vi "Is_it_a_Results_File.vi"(0 "character string":string) -> (1 "Contain DB Header Info":bool, 2 "Header String":string, 3 "Results File?":bool)   [LabVIEW 2020]
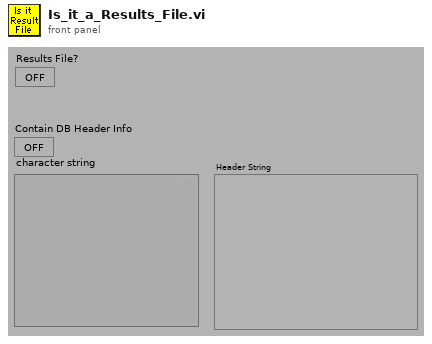
[diagram p1: front panel]
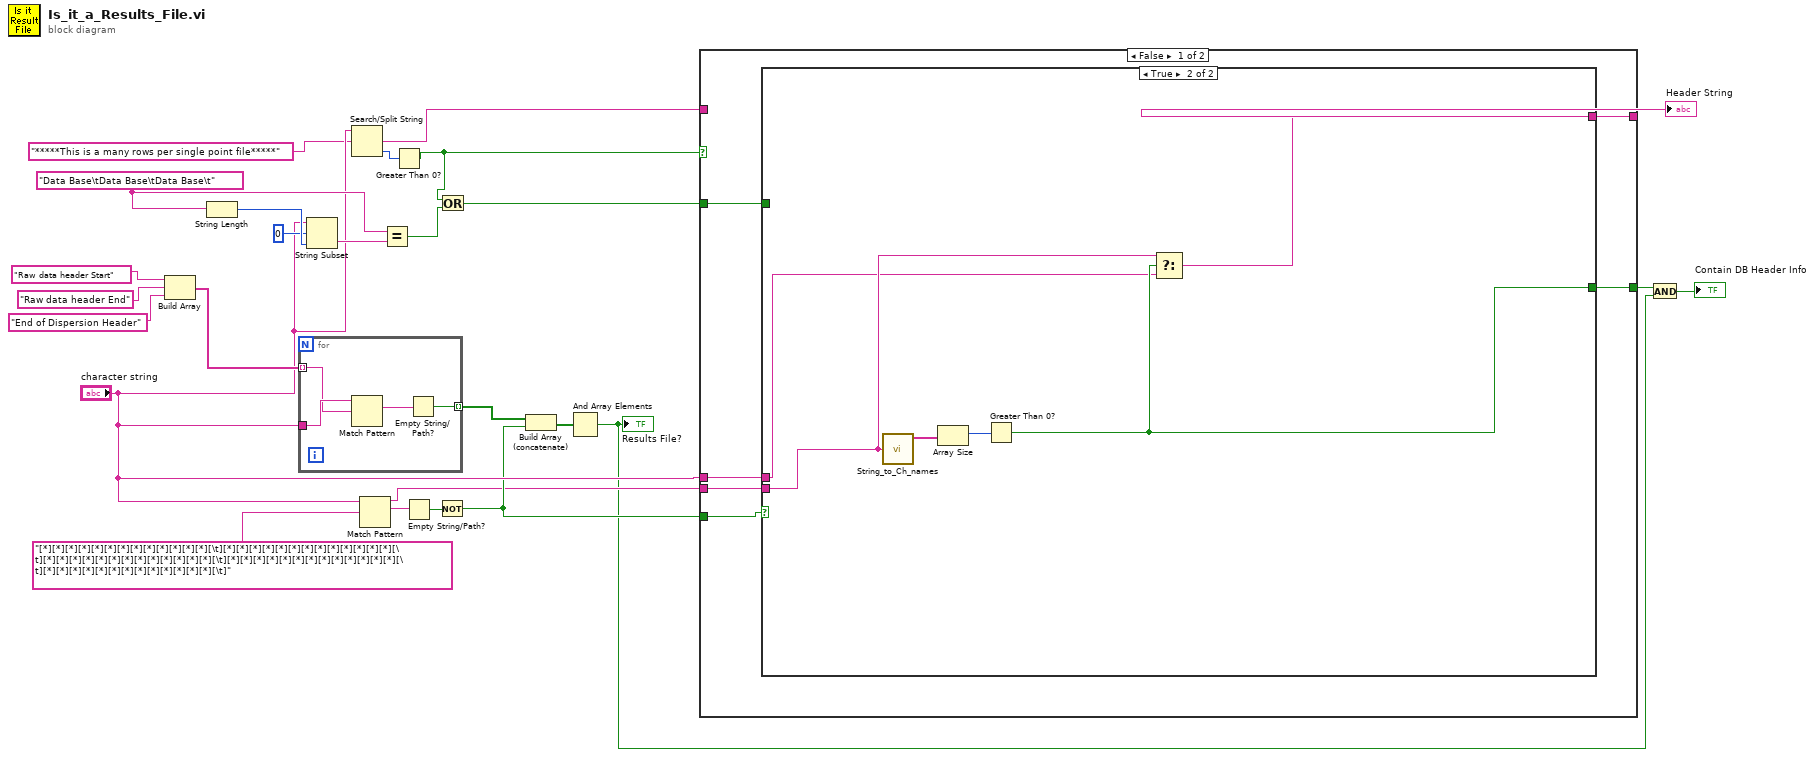
[diagram p0: block diagram]
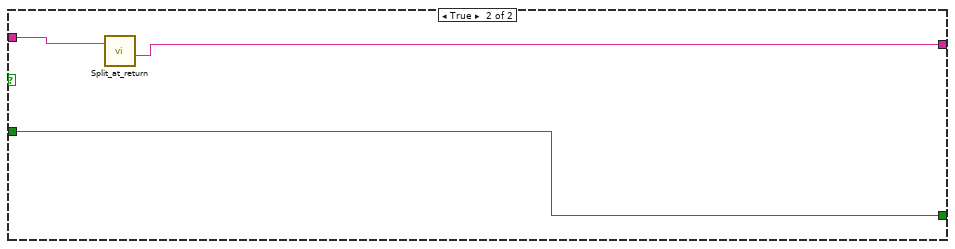
[diagram p3: hidden frame]
diagram:
  w14 = "Data Base\tData Base\tData Base\t"
  n1 = Build Array("Raw data header Start", "Raw data header End", "End of Dispersion Header") -> (w24:string[])
  n2 = String Length(string=w14) -> (length=w17:i32)
  n3 = for {
    tunnel: "character string" -> [w30]
    tunnel: w24 -> [w29] mode=indexing
    tunnel: [w27] -> w21 mode=indexing
    n4 = Match Pattern(string=w30, regular expression=w29) -> (match substring=w28:string)  [unwired: 4 out]
    n5 = Empty String/Path?(string/path=w28) -> (empty?=w27:bool)
  }
  n6 = String Subset(string="character string", offset (0)=0, length (rest)=w17) -> (substring=w15:string)
  n7 = Search/Split String(string="character string", search string/char (-)="*****This is a many rows per single point file*****") -> (match + rest of string=w12:string, offset of match=w8:i32)  [unwired: 2 out]
  n8 = Match Pattern(string="character string", regular expression="[*][*][*][*][*][*][*][*][*][*][*][*][*][\t][*][*][*][*][*][*][*][*][*][*][*][*][*][\t][*][*][*][*][*][*][*][*][*][*][*][*][*][\t][*][*][*][*][*][*][*][*][*][*][*][*][*][\t][*][*][*][*][*][*][*][*][*][*][*][*][*][\t]" ("String")) -> (before substring=w5:string, match substring=w23:string)  [unwired: 3 out]
  n9 = Equal?(x=w14, y=w15) -> (x = y?=w13:bool)
  n10 = Greater Than 0?(x=w8) -> (x > 0?=w7:bool)
  n11 = Empty String/Path?(string/path=w23) -> (empty?=w22:bool)
  n12 = Not(x=w22) -> (.not. x?=w6:bool)
  n13 = Or(x=w7, y=w13) -> (x .or. y?=w1:bool)
  n14 = Build Array (concatenate)(w21, w6) -> (w20:bool[])
  n15 = And Array Elements(Boolean array=w20) -> (logical AND=w3:bool)
  "Results File?" <- w3
  n16 = case shown="False" w7 {
    tunnel: w12 -> [_ w47]
    tunnel: [w34 w46] -> w11
    tunnel: "character string" -> [w35 _]
    tunnel: w6 -> [w36 _]
    tunnel: w5 -> [w33 _]
    tunnel: [w32 w45] -> w2
    tunnel: w1 -> [w31 w45]
    frame False {
      n17 = case shown="True" w36 {
        tunnel: w35 -> [w38 w40]
        tunnel: [w38 w39] -> w34
        tunnel: w33 -> [_ w41]
        tunnel: [w37 w42] -> w32
        tunnel: w31 -> [w37 _]
        frame False {
        }
        frame True {
          n18 = call "String_to_Ch_names.vi"("Spreadsheet string"=w41) -> ("Ch names"=w44:string[])  [unwired: 3 out]
          n19 = Array Size(array=w44) -> (size(s)=w43:i32)
          n20 = Greater Than 0?(x=w43) -> (x > 0?=w42:bool)
          n21 = Select(t=w41, s=w42, f=w40) -> (s? t:f=w39:string)
        }
      }
    }
    frame True {
      n22 = call "Split_at_return.vi"("String"=w47) -> ("after substring"=w46:string)  [unwired: 1 in, 3 out]
    }
  }
  "Header String" <- w11
  n23 = And(x=w2, y=w3) -> (x .and. y?=→"Contain DB Header Info":bool)
